vi "KHE - Root Directory.vi"() -> (0 "Project Root Directory":path)   [LabVIEW 2016]
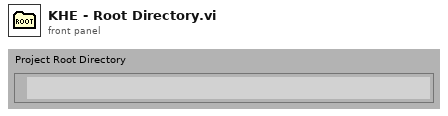
[diagram p1: front panel]
types:
  T1 = enum32{"invalid app kind", "Development System", "Run Time System", "Student Edition", "Embedded LabVIEW", "Evaluation", "Custom"}
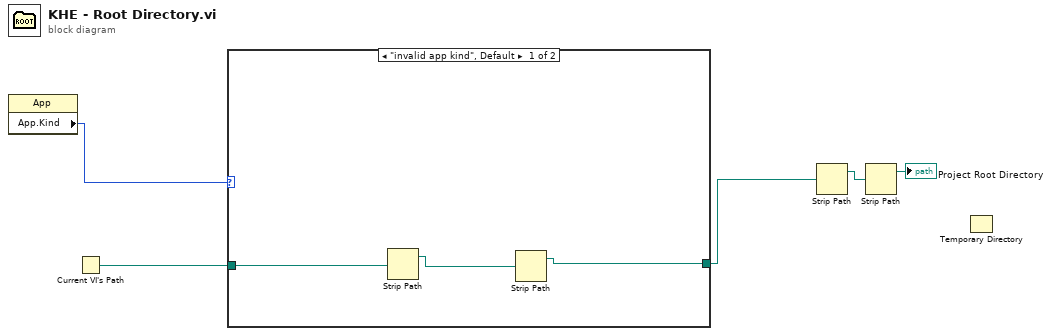
[diagram p0: block diagram]
diagram:
  n1 = property class="App"() -> ("App.Kind"=w3:T1)  [unwired: 2 in, 2 out]
  n2 = Current VI's Path() -> (path=w2:path)
  n3 = case shown="\"invalid app kind\", Default" w3 {
    tunnel: w2 -> [w8 w9]
    tunnel: [w6 w9] -> w1
    frame "invalid app kind", Default {
      n4 = Strip Path(path=w8) -> (stripped path=w7:path)  [unwired: 1 out]
      n5 = Strip Path(path=w7) -> (stripped path=w6:path)  [unwired: 1 out]
    }
    frame "Development System" {
    }
  }
  n6 = Strip Path(path=w1) -> (stripped path=w5:path)  [unwired: 1 out]
  n7 = Strip Path(path=w5) -> (stripped path=→"Project Root Directory":path)  [unwired: 1 out]
  n8 = Temporary Directory() -> ()  [unwired: 1 out]
